vi "Tclock_to_Unix_time.vi"(9 "Unix epoch zerotime (nanoseconds)":u64, 11 "Timestamps (seconds from T0)":dbl[](array[numeric]) format="%#.25g") -> (3 "Unix Timestamps (nanoseconds)":u64[](array[numeric]))   [LabVIEW 2021, in "Ring Buffer Strict Accessor.lvlib" / "Unix time epoch.lvlib"]
uses:
  Unix time epoch.lvlib
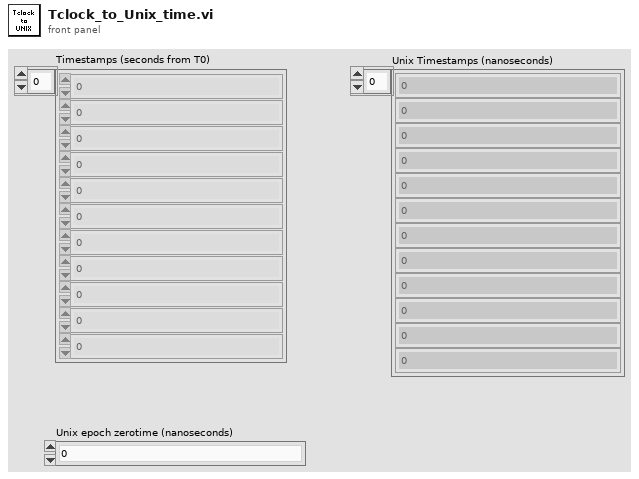
[diagram p1: front panel]
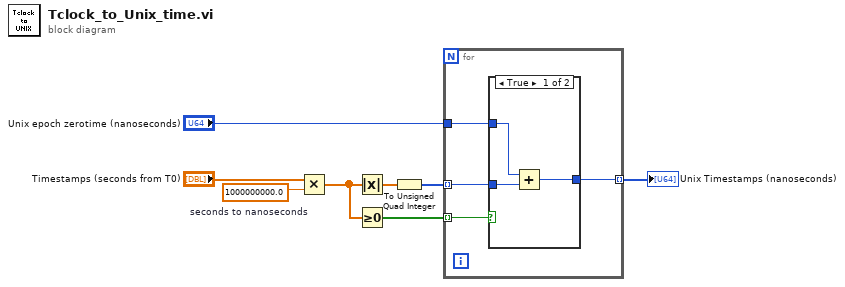
[diagram p0: block diagram]
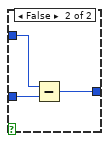
[diagram p2: hidden frame]
diagram:
  w8 = 1000000000.0  # seconds to nanoseconds
  n1 = Multiply(x="Timestamps (seconds from T0)", y=w8) -> (x*y=w3:dbl[])
  n2 = Absolute Value(x=w3) -> (abs(x)=w2:dbl[])
  n3 = Greater Or Equal To 0?(x=w3) -> (x >= 0?=w6:bool[])
  n4 = To Unsigned Quad Integer(1:w2) -> (0:w4:u64[])
  n5 = for {
    tunnel: [w12] -> w1 mode=indexing
    tunnel: "Unix epoch zerotime (nanoseconds)" -> [w11]
    tunnel: w4 -> [w10] mode=indexing
    tunnel: w6 -> [w9] mode=indexing
    n6 = case shown="True" w9 {
      tunnel: [w15 w18] -> w12
      tunnel: w11 -> [w14 w17]
      tunnel: w10 -> [w13 w16]
      frame True {
        n7 = Add(x=w14, y=w13) -> (x+y=w15:u64)
      }
      frame False {
        n8 = Subtract(x=w17, y=w16) -> (x-y=w18:u64)
      }
    }
  }
  "Unix Timestamps (nanoseconds)" <- w1
